vi "Initial States.vi"(8 "error in":errorcluster, 10 "States":string[](array[string]), 11 "Test Case In":refnum<class "History Tests.lvclass">) -> (0 "error out":errorcluster, 2 "Expected Undo Stack":string[](array[string]), 3 "Test Case Out":refnum<class "History Tests.lvclass">, 4 "Current State":string)   [LabVIEW 2020, in "History Tests.lvclass"]
uses:
  History Tests.lvclass
  History Tests.lvclass/History Tests.ctl
  resource/plugins/NIIconEditor/History/History/History.lvclass
  7911fddc-fa75-4b8f-ab0b-e19a35acb203.vi
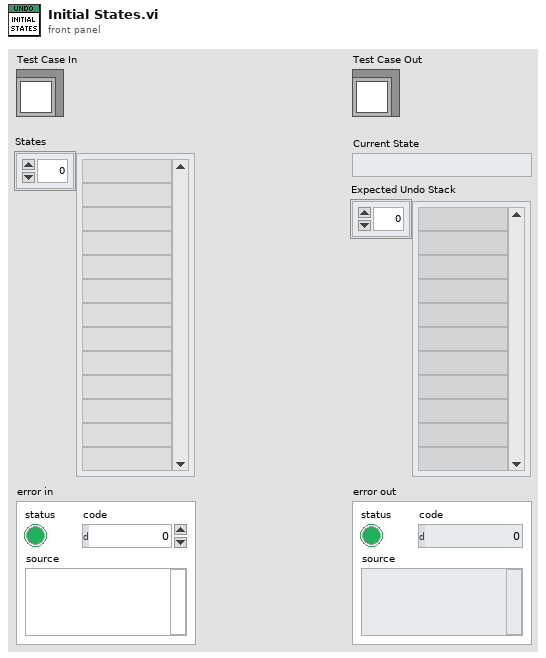
[diagram p1: front panel]
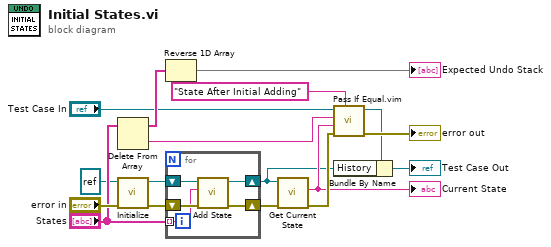
[diagram p0: block diagram]
diagram:
  n1 = Delete From Array(array="States") -> (deleted portion=w11:string, array with subset deleted=w12:string[])  [unwired: 2 in]
  n2 = call "Initialize.vi"("error in"="error in", "menu reference"=refnum<k9> refnum) -> ("error out"=w16:errorcluster, "History"=w5:refnum<class "History.lvclass">)  [unwired: 8 in]
  n3 = Reverse 1D Array(array=w12) -> (reversed array=→"Expected Undo Stack":string[])
  n4 = for {
    tunnel: "States" -> [w18] mode=indexing
    shift-right: [w21] -> w14
    shift-left: w16 -> [w22]
    shift-right: [w19] -> w2
    shift-left: w5 -> [w20]
    n5 = call "Add State.vi"("error in"=w22, "State"=w18, "History in"=w20) -> ("error out"=w21:errorcluster, "History out"=w19:refnum<class "History.lvclass">)  [unwired: 7 in]
  }
  n6 = call "Get Current State.vi"("error in"=w14, "History"=w2) -> ("error out"=w13:errorcluster, "Current State"=w7:string)  [unwired: 7 in, 1 out]
  "Current State" <- w7
  n7 = call "Pass If Equal.vim"("Description"="State After Initial Adding", "error in (no error)"=w13, "Actual"=w7, "Expected"=w11, "LUnit Test Case In"="Test Case In") -> ("error out"=→"error out":errorcluster, "LUnit Test Case Out"=w3:refnum<class "History Tests.lvclass">)  [unwired: 5 in]
  n8 = Bundle By Name(cluster=w3, "History"=w2) -> (→"Test Case Out":refnum<class "History Tests.lvclass">)
